vi "Rotation.vi"(0 "Time":dbl, 1 "Speed (ft/sec)":dbl) -> ()   [LabVIEW 2012]
uses:
  <vilib>/Rock Robotics/WPI/RobotDrive/WPI_RobotDriveGetSetRefNum.vi
  <vilib>/Rock Robotics/WPI/RobotDrive/WPI_RobotDriveMecanumDrive_Cartesian.vi
panel:
  # "Rate  =/- 1.00"
  # "Sconds"
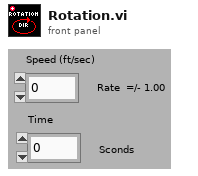
[diagram p1: front panel]
types:
  T1 = typedef "WPI_RobotDriveDevRef.ctl" = cluster{"DevStatus":errorcluster, "Motors[]":T2[], "Square Inputs":bool, "Max Output":dbl, "Isochronous":bool}
  T2 = typedef "WPI_MotorControlDeviceRef.ctl" = cluster{"DeviceStatus":errorcluster, "Type":enum16{"PWM", "CAN"}, "PWM":cluster{"Digital Module":T3, "PWM Channel":T4, "DeadBand":T5}, "CAN":cluster{"Device Number":u8, "Control Mode":T6, "Semaphore":T7, "Max Vout":dbl}, "Invert":bool, "TransformRef":T8, "InvTransformRef":T8}
  T3 = typedef "FPGA_TypedefDigitalModule.ctl" = enum16{"Digital Module 1", "Digital Module 2"}
  T4 = typedef "FPGA_DIOPWMChannel.ctl" = enum8{"PWM 1", "PWM 2", "PWM 3", "PWM 4", "PWM 5", "PWM 6", "PWM 7", "PWM 8", "PWM 9", "PWM 10", "Invalid"}
  T5 = typedef "WPI_PWMDeadband.ctl" = cluster{"Name":string, "maxPositivePwm":i32, "minPositivePwm":i32, "centerPwm":i32, "maxNegativePwm":i32, "minNegativePwm":i32, "angularRange":u16}
  T6 = typedef "WPI_CANJaguar_ControlMode.ctl" = enum8{"Percent VBus", "Current", "Speed", "Position", "Voltage"}
  T7 = typedef "Semaphore RefNum" = refnum<k1>
  T8 = typedef "WPI_PWMTransform_ConPane.ctl" = refnum<vi>
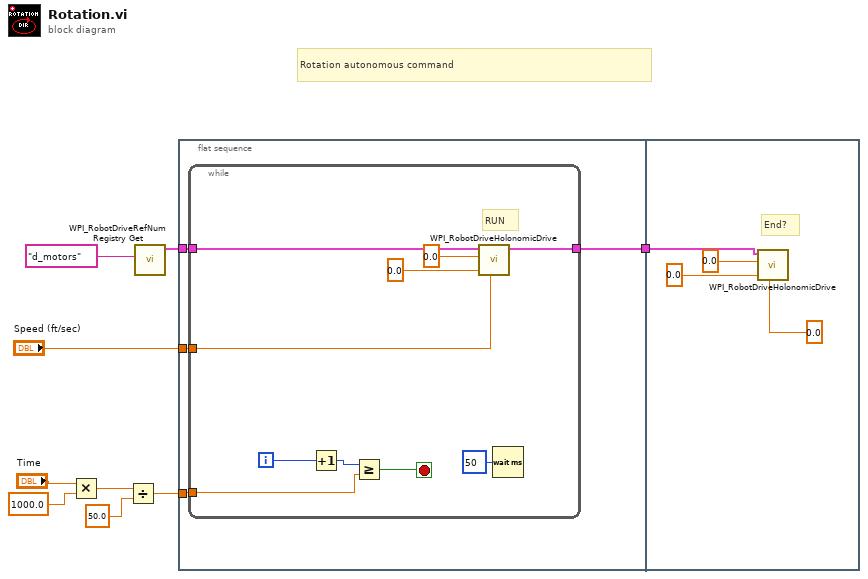
[diagram p0: block diagram]
diagram:
  # "Rotation autonomous command"
  n1 = Multiply(x="Time", y=1000.0) -> (x*y=w4:dbl)
  n2 = Divide(x=w4, y=50.0) -> (x/y=w2:dbl)
  n3 = call <vilib>:"WPI_RobotDriveRefNum Registry Get.vi"("refnum name"="d_motors") -> ("RobotDriveDevRef"=w8:T1)  [unwired: 1 in, 9 out]
  n4 = flat-sequence {
    tunnel: w8 -> [w13]
    tunnel: "Speed (ft/sec)" -> [w12]
    tunnel: w2 -> [w11]
    tunnel: [w10] -> w1
    tunnel: w1 -> [w25]
    frame #0 {
      n5 = while {
        tunnel: w13 -> [w22]
        tunnel: w11 -> [w18]
        tunnel: w12 -> [w16]
        tunnel: [w14] -> w10
        i -> [w21]
        stop <- w19 stop-if-true
        # "RUN"
        n6 = Increment(x=w21) -> (x+1=w20:i32)
        n7 = Greater Or Equal?(x=w20, y=w18) -> (x >= y?=w19:bool)
        n8 = call-poly <vilib>:"WPI_RobotDriveHolonomicDrive.vi"("Rotation"=w16, "Y"=0.0 ("Rotation"), "X"=0.0 ("Magnitude"), "RobotDriveDevRef"=w22) -> ("RobotDriveDevRef"=w14:T1)  [unwired: 5 in, 2 out]
        n9 = Wait (ms)(milliseconds to wait=u32 50) -> ()  [unwired: 1 out]
      }
    }
    frame #1 {
      # "End?"
      n10 = call-poly <vilib>:"WPI_RobotDriveHolonomicDrive.vi"("Rotation"=0.0, "Y"=0.0 ("Rotation"), "X"=0.0 ("Magnitude"), "RobotDriveDevRef"=w25) -> ()  [unwired: 5 in, 3 out]
    }
  }
